vi "Actor Core.vi"(8 "error in":errorcluster, 11 "UI_Actor in":refnum<class "UI_Actor.lvclass">) -> (0 "error out":errorcluster, 3 "Actor out":refnum<class "Actor.lvclass">)   [LabVIEW 2020, in "UI_Actor.lvlib" / "UI_Actor.lvclass"]
doc: "(<B>Filename</B>: Actor Framework.lvlib:Actor.lvclass:Actor Core.vi)\n\nReceives messages to the actor, reacts to them, and initiates any error handling that may shut the actor down.\n\nDescendant classes may override this VI to append parallel tasks for the actor to complete while it handles messages. Overrides use the Call Parent Method node."
uses:
  UI_Actor.lvclass
  D:/Projets/STEP AT/UI Actor/support/Actor Framework.lvlibp/1abvi3w/vi.lib/ActorFramework/Actor/Actor.lvclass
  support/Actor Framework.lvlibp/1abvi3w/vi.lib/ActorFramework/Actor/Actor.lvclass
  support/Actor Framework.lvlibp/1abvi3w/vi.lib/ActorFramework/Message Enqueuer/Message Priority.ctl
  UI_Actor.lvclass/UI_Actor.ctl
  support/Actor Framework.lvlibp/1abvi3w/vi.lib/ActorFramework/Message Enqueuer/Enqueue.vi
  UI_Actor Messages/priv_Store.UI.Ref Msg/priv_Store.UI.Ref Msg.lvclass
  support/Actor Framework.lvlibp/1abvi3w/vi.lib/ActorFramework/Message Enqueuer/Message Enqueuer.lvclass
panel:
  # "UI ACTOR PARENT\n\nINTERFACE DE TEST"
  # "Tu as peut etre oublier d'override le Core mon bonhomme"
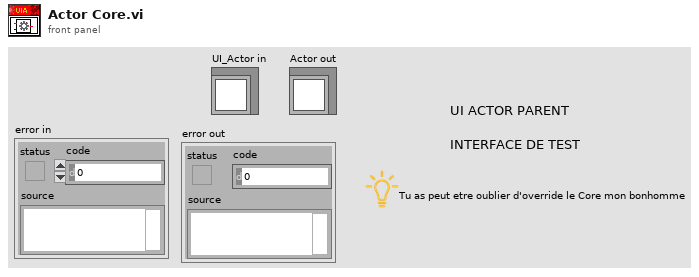
[diagram p1: front panel]
types:
  T1 = typedef "Actor Framework.lvlibp/Message Enqueuer.lvclass/Message Priority.ctl" = enum16{"Low", "Normal", "High"}
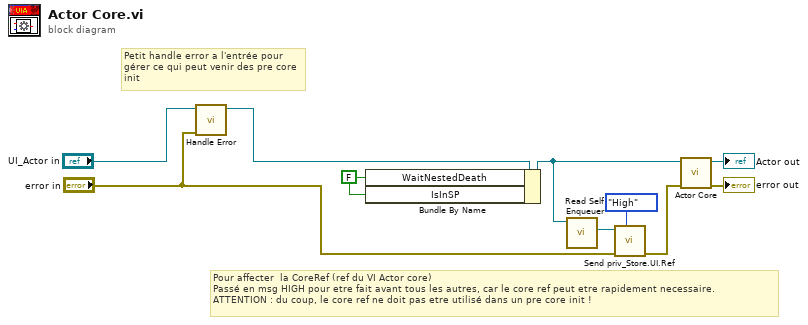
[diagram p0: block diagram]
diagram:
  w5 = FALSE ("WaitNestedDeath")
  # "Petit handle error a l'entrée pour gérer ce qui peut venir des pre core init"
  # "Pour affecter  la CoreRef (ref du VI Actor core)\nPassé en msg HIGH pour etre fait avant tous les autres, car le core ref peut etre rapidement necessaire.\nATTENTION : du coup, le core ref ne doit pas etre utilisé dans un pre core init !"
  n1 = call-dynamic "Handle Error.vi"("error in (no error)"="error in", "UI_Actor in"="UI_Actor in") -> ("UI_Actor out"=w1:refnum<class "UI_Actor.lvclass">)  [unwired: 7 in, 2 out]
  n2 = Bundle By Name(cluster=w1, "WaitNestedDeath"=w5, "IsInSP"=w5) -> (w6:refnum<class "UI_Actor.lvclass">)
  n3 = call "Read Self Enqueuer.vi"("Actor"=w6) -> ("Self Enqueuer"=w8:refnum<class "Message Enqueuer.lvclass">)  [unwired: 10 in]
  n4 = call "Send priv_Store.UI.Ref.vi"("Message Priority (Normal)"=Message_Priority."High" ("Message Priority"), "error in (no error)"="error in", "Message Enqueuer"=w8) -> ("error out"=w10:errorcluster)  [unwired: 7 in, 1 out]
  n5 = call-parent "Actor Core.vi"("error in"=w10, "Actor in"=w6) -> ("error out"=→"error out":errorcluster, "Actor out"=→"Actor out":refnum<class "Actor.lvclass">)  [unwired: 8 in]
